vi "Status Close.vi"(8 "error in":errorcluster, 11 "Status Reference":T1) -> (0 "error out":errorcluster)   [LabVIEW 2021, in "Status.lvlib"]
uses:
  Status.lvlib
  Ctl/control.ctl
  Ctl/State.ctl
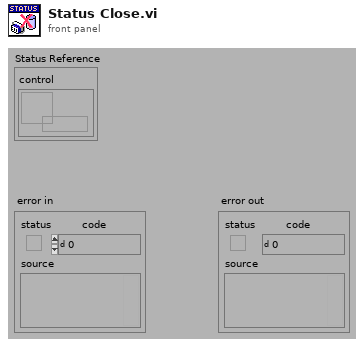
[diagram p1: front panel]
types:
  T1 = typedef "Status.lvlib/control.ctl" = cluster{"control":refnum<data-value>}
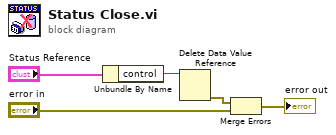
[diagram p0: block diagram]
diagram:
  n1 = Unbundle By Name("Status Reference") -> ("control"=w3:refnum<data-value>)
  n2 = Delete Data Value Reference(data value reference=w3) -> (error out=w4:errorcluster)  [unwired: 1 in, 1 out]
  n3 = Merge Errors(w4, "error in") -> (→"error out":errorcluster)
